vi "Periodic Tasks.vi"(8 "error in":errorcluster) -> ()   [LabVIEW 2018]
doc: "This VI runs in parallel to other tasks. It can contain as many user-defined periodic loops as you need. These can carry out PID or other sorts of timed response."
uses:
  <vilib>/Rock Robotics/WPI/DriverStation/WPI_DriverStationRobotMode2.ctl
  Cargo_motor_states.ctl
  control_states.ctl
  <vilib>/Rock Robotics/WPI/ThirdParty/Phoenix-LabVIEW/Motor Controller/Controls/CTRE_Phoenix_MotorControl_ControlMode.ctl
  GP_states.ctl
  <vilib>/Rock Robotics/WPI/Relay/WPI_RelayValue.ctl
  <vilib>/Analysis/baseanly.llb/Mean (DBL).vi
  <vilib>/Rock Robotics/Network Tables/NT Read Boolean.vi
  Robot Global Data.vi
  <vilib>/Rock Robotics/Network Tables/NT Read Numeric Array.vi
  <vilib>/Rock Robotics/Network Tables/NT Write Numeric Array.vi
  <vilib>/Rock Robotics/Network Tables/NT Write Boolean Array.vi
  <vilib>/Rock Robotics/Network Tables/NT Write Number.vi
  <vilib>/Rock Robotics/Network Tables/NT Read Number.vi
  <vilib>/addons/control/pid/pid.llb/PID (DBL).vi
  drivers/ADIS16470 IMU/ADIS16470_IMU.lvlib
  <vilib>/addons/control/pid/NI_PID_pid.lvlib
  <vilib>/Analysis/NI_AALBase.lvlib
panel:
  out "Robot Mode":T1
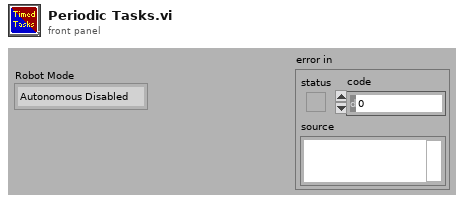
[diagram p1: front panel]
types:
  T1 = typedef "WPI_DriverStationRobotMode2.ctl" = enum16{"Autonomous Disabled", "Autonomous Enabled", "Teleop Disabled", "Teleop Enabled", "Disconnected", "Finish", "Test Disabled", "Test Enabled", "Emergency Stopped"}
  T2 = enum16{"open", "replace", "create", "open or create", "replace or create", "replace or create with confirmation"}
  T3 = typedef "Cargo_motor_states.ctl" = enum16{"Idle", "Intake", "Shoot"}
  T4 = typedef "ADIS16470_IMU.lvlib/ADI_IMU_ADIS16470_IMUDevRef.ctl" = cluster{"DevStatus":errorcluster, "Handle":i32, "SPI Bus":T5, "Device Found":bool, "Device Ready":bool, "Serial":u16, "Bytes Per Sample":u16, "Calibrate On Open?":bool}
  T5 = typedef "spi_bus.ctl" = enum16{"SPI On-Board, CS0", "SPI On-Board, CS1", "SPI On-Board, CS2", "SPI On-Board, CS3", "SPI MXP", "Invalid"}
  T6 = typedef "WPI_DigitalInputDevRef.ctl" = cluster{"DevStatus":errorcluster, "DIO Channel":T7}
  T7 = typedef "FPGA_DIOChannel.ctl" = enum8{"DIO 0", "DIO 1", "DIO 2", "DIO 3", "DIO 4", "DIO 5", "DIO 6", "DIO 7", "DIO 8", "DIO 9", "DIO MXP 0", "DIO MXP 1", "DIO MXP 2", "DIO MXP 3", "DIO MXP 4", "DIO MXP 5", "DIO MXP 6", "DIO MXP 7", "DIO MXP 8", "DIO MXP 9", "DIO MXP 10", "DIO MXP 11", "DIO MXP 12", "DIO MXP 13", "DIO MXP 14", "DIO MXP 15", "SPI Port CS1", "SPI Port CS2", "SPI Port CS3", "SPI Port MISO", "SPI Port MOSI", "Invalid"}
  T8 = typedef "WPI_PotentiometerDevRef.ctl" = cluster{"DevStatus":errorcluster, "Analog Channel":T9, "Invert Output":bool}
  T9 = typedef "FPGA_AIChannel.ctl" = enum8{"AI 0", "AI 1", "AI 2", "AI 3", "AI MXP 0", "AI MXP 1", "AI MXP 2", "AI MXP 3", "Invalid"}
  T10 = typedef "WPI_RelayDevRef.ctl" = cluster{"DevStatus":errorcluster, "Relay Channel":T11, "Relay Direction":T12}
  T11 = typedef "FPGA_DIORelayChannel.ctl" = enum8{"Relay 0", "Relay 1", "Relay 2", "Relay 3", "Invalid"}
  T12 = typedef "WPI_RelayDirection.ctl" = enum16{"Both directions", "Forward only", "Reverse only"}
  T13 = typedef "WPI_MotorControlDeviceRef.ctl" = cluster{"DeviceStatus":errorcluster, "Type":T14, "PWM":cluster{"PWM Channel":T15, "DeadBand":T16}, "CAN":cluster{"Device Number":u8, "SetOutput VI Ref":variant, "GetOutput VI Ref":variant, "Enable VI Ref":variant, "Disable VI Ref":variant, "Data":variant}, "Invert":bool, "DIO PWM":cluster{"PWM \"Enable\" Channel":T15, "DIOChannel":T7, "PWM Rate":dbl}}
  T14 = typedef "WPI_MotorControlType.ctl" = enum16{"PWM", "CAN", "DIO PWM"}
  T15 = typedef "FPGA_DIOPWMChannel.ctl" = enum8{"PWM 0", "PWM 1", "PWM 2", "PWM 3", "PWM 4", "PWM 5", "PWM 6", "PWM 7", "PWM 8", "PWM 9", "PWM MXP 0", "PWM MXP 1", "PWM MXP 2", "PWM MXP 3", "PWM MXP 4", "PWM MXP 5", "PWM MXP 6", "PWM MXP 7", "PWM MXP 8", "PWM MXP 9", "Invalid"}
  T16 = typedef "WPI_PWMDeadband.ctl" = cluster{"Name":string, "maxPositivePwm":i32, "minPositivePwm":i32, "centerPwm":i32, "maxNegativePwm":i32, "minNegativePwm":i32, "angularRange":u16}
  T17 = typedef "CTRE_Phoenix_MotorControl_ControlMode.ctl" = u16
  T18 = typedef "WPI_RelayValue.ctl" = enum16{"Off", "On", "Forward", "Reverse"}
  T19 = typedef "control_states.ctl" = enum16{"disable", "PID", "motor"}
  T20 = typedef "GP_states.ctl" = enum16{"Home", "AutoHome", "Hatch", "Ground"}
  T21 = cluster{"dorsalPID[0]":dbl, "dorsalPID[1]":dbl, "dorsalPID[2]":dbl}
  T22 = cluster{"fourbarPID[0]":dbl, "fourbarPID[1]":dbl, "fourbarPID[2]":dbl}
  T23 = cluster{"X Angle":dbl, "Y Angle":dbl, "Z Angle":dbl}
  T24 = cluster{"X Gyro":dbl, "Y Gyro":dbl, "Z Gyro":dbl, "X Accel":dbl, "Y Accel":dbl, "Z Accel":dbl, "Temp":dbl}
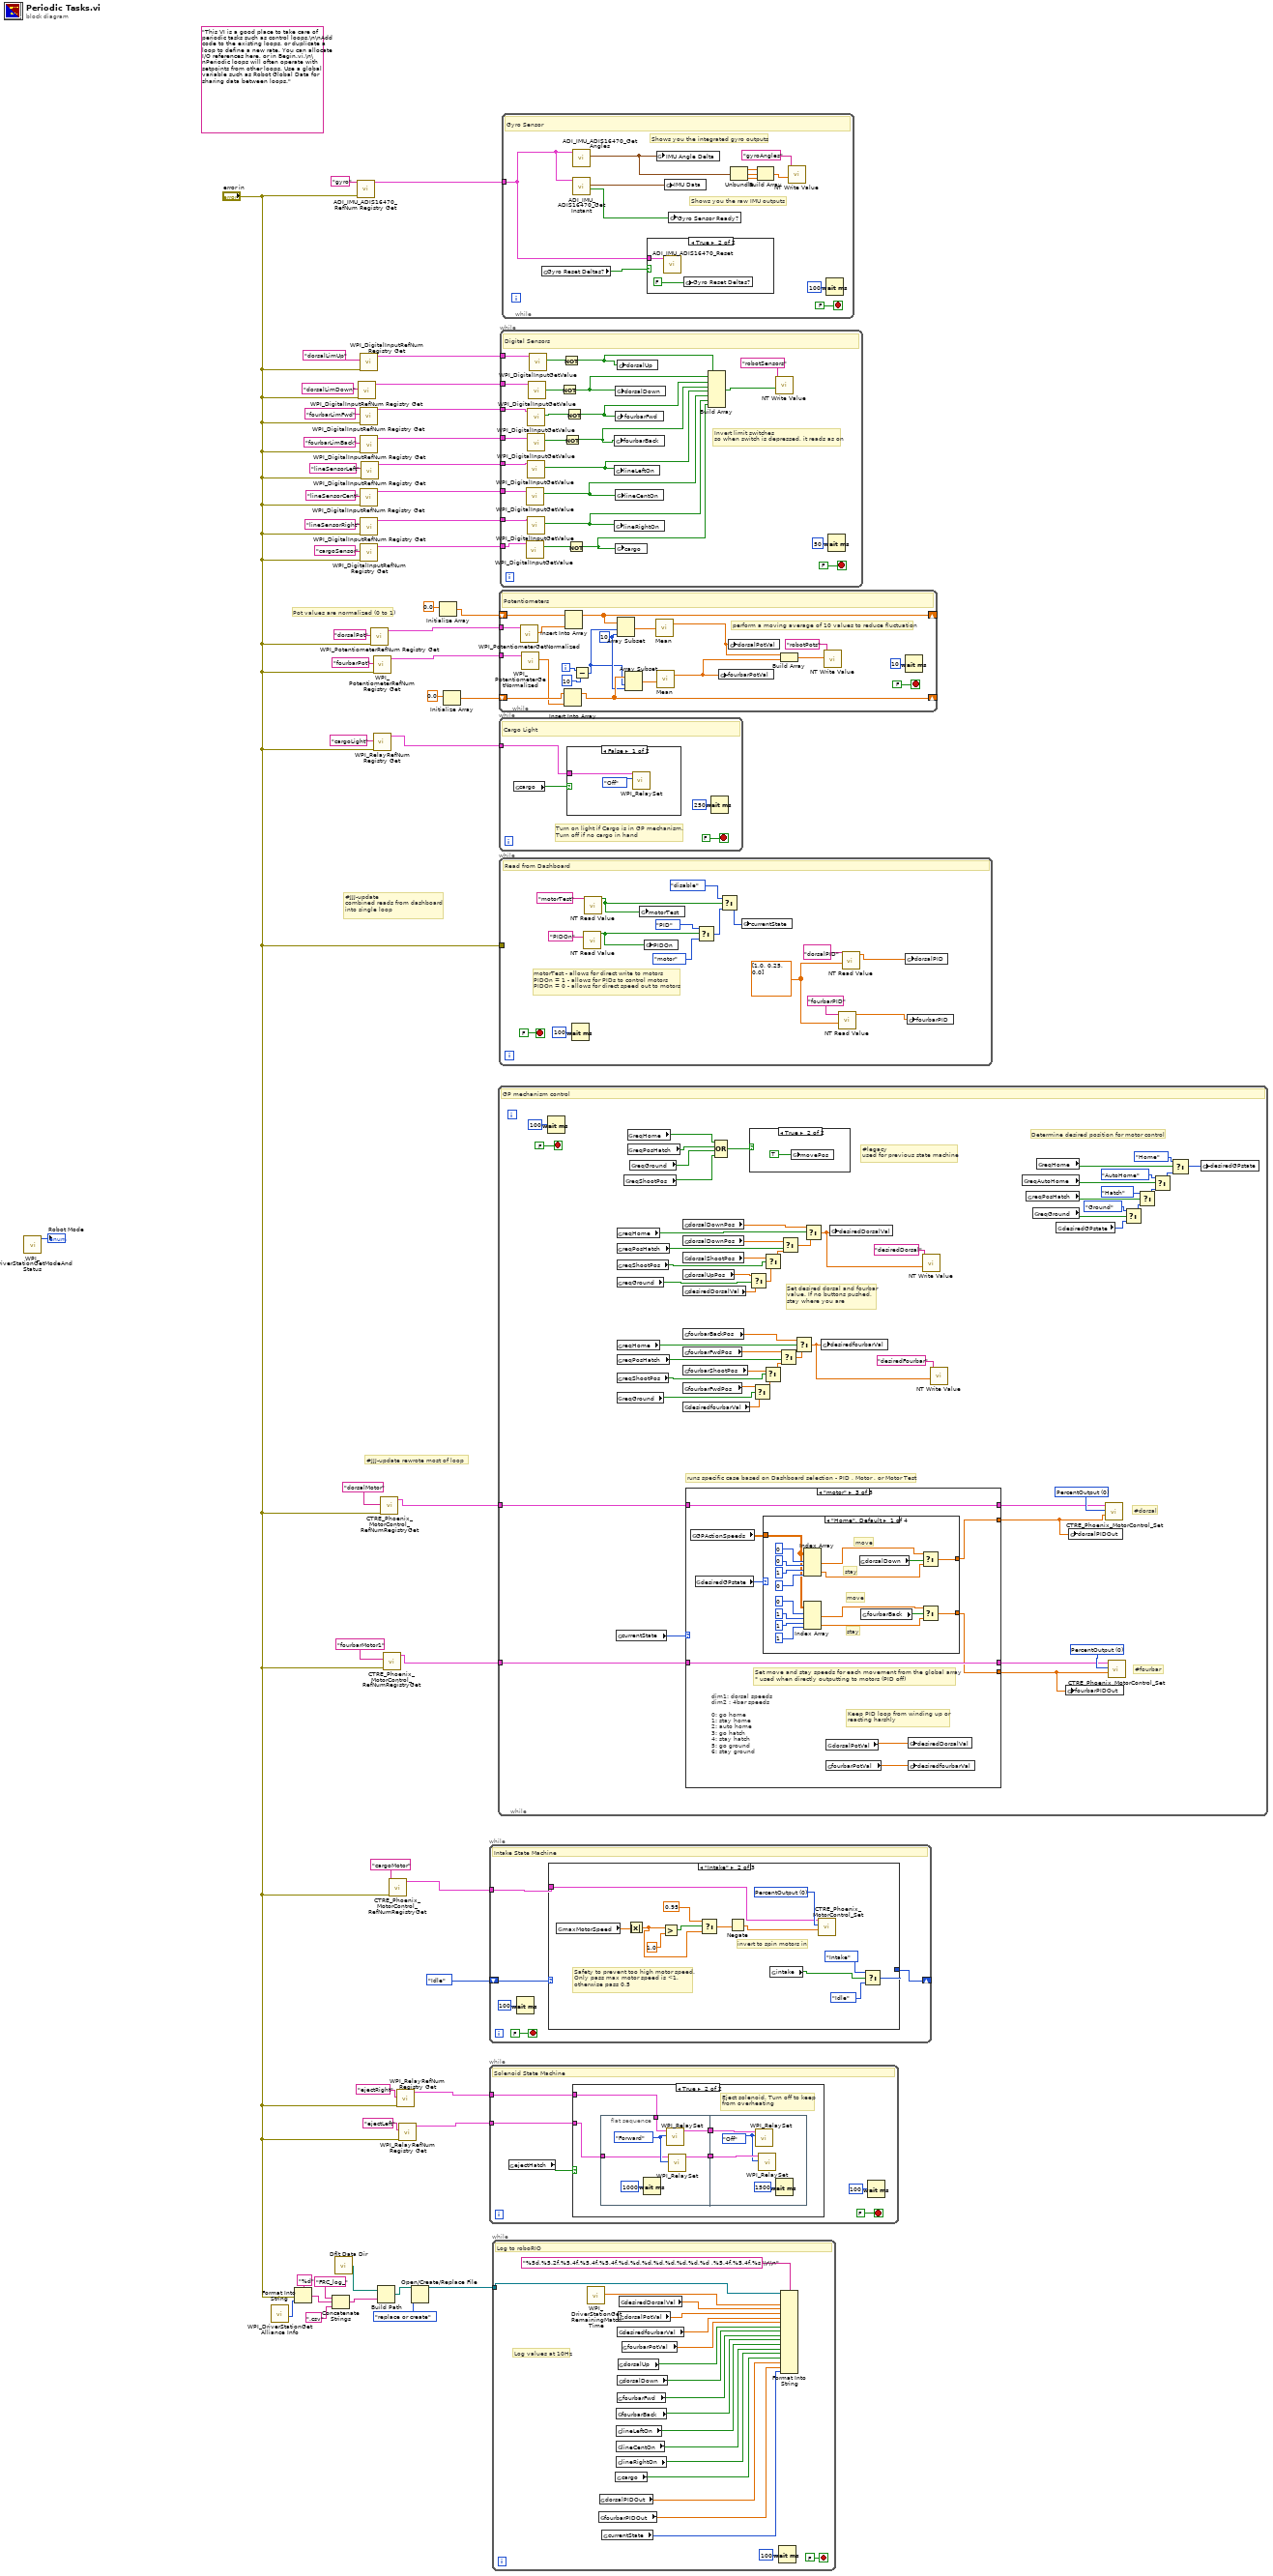
[diagram p0: block diagram]
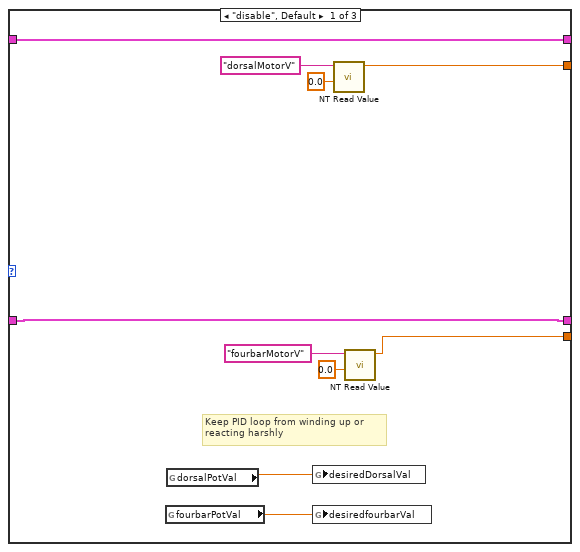
[diagram p2: hidden frame]
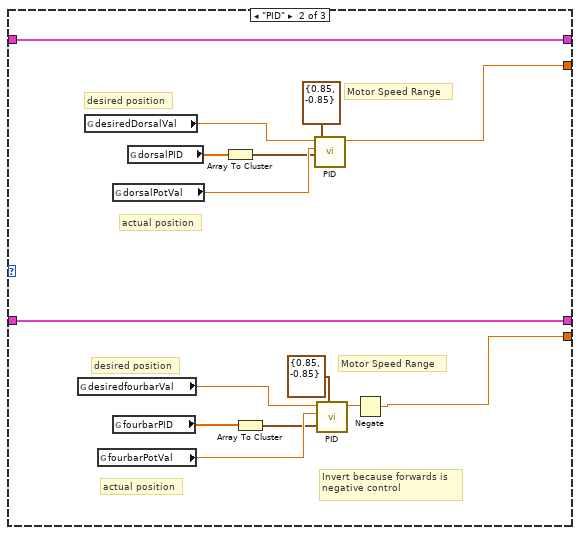
[diagram p3: hidden frame]
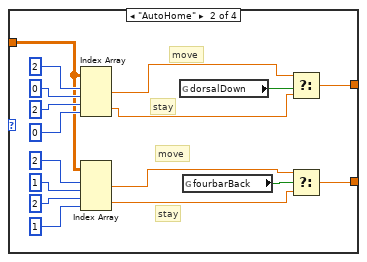
[diagram p4: hidden frame]
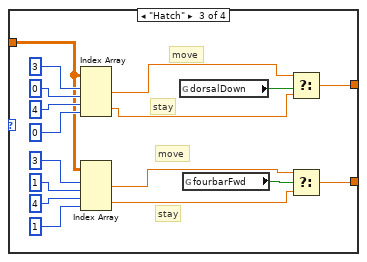
[diagram p5: hidden frame]
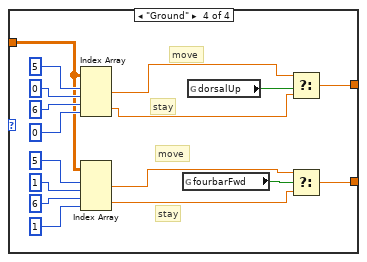
[diagram p6: hidden frame]
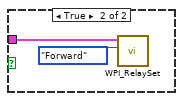
[diagram p8: hidden frame]
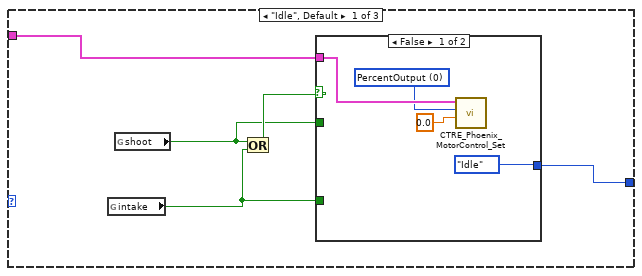
[diagram p10: hidden frame]
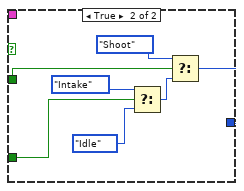
[diagram p11: hidden frame]
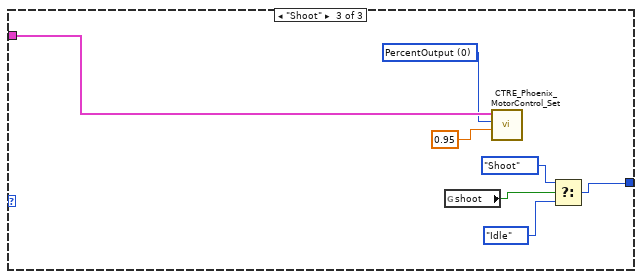
[diagram p12: hidden frame]
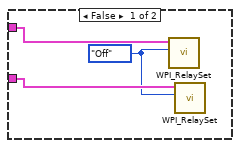
[diagram p13: hidden frame]
diagram:
  (unwired) "This VI is a good place to take care of periodic tasks such as control loops.\n\nAdd code to the existing loops, or duplicate a loop to define a new rate. You can allocate I/O references here, or in Begin.vi.\n\nPeriodic loops will often operate with setpoints from other loops. Use a global variable such as Robot Global Data for sharing data between loops."
  # "#JJJ-update rewrote most of loop"
  # "#JJJ-update\ncombined reads from dashboard\ninto single loop"
  # "Pot values are normalized (0 to 1)"
  n1 = call <vilib>:"WPI_DriverStationGetModeAndStatus.vi"() -> ("Robot Mode"=→"Robot Mode":T1)  [unwired: 10 in, 1 out]
  n2 = call <vilib>:"WPI_DriverStationGet Alliance Info.vi"() -> ("Match Number"=w9:u16)  [unwired: 6 in, 5 out]
  n3 = Format Into String(format string="%d", error in="error in", w9) -> (resulting string=w8:string)  [unwired: 1 in, 1 out]
  n4 = Concatenate Strings("FRC_log_", w8, ".csv" ("string")) -> (w12:string)
  n5 = call <vilib>:"Dflt Data Dir.vi"() -> ("App:Default Data Directory"=w16:path)
  n6 = call "ADI_IMU_ADIS16470_RefNum Registry Get.vi"("error in (no error)"="error in", "refnum name"="gyro") -> ("ADI IMU DevRef"=w51:T4)  [unwired: 8 in, 1 out]
  n7 = call <vilib>:"WPI_DigitalInputRefNum Registry Get.vi"("error in (no error)"="error in", "refnum name"="dorsalLimDown") -> ("DigitalInputDevRef"=w48:T6)  [unwired: 8 in, 1 out]
  n8 = call <vilib>:"WPI_DigitalInputRefNum Registry Get.vi"("error in (no error)"="error in", "refnum name"="dorsalLimUp") -> ("DigitalInputDevRef"=w49:T6)  [unwired: 8 in, 1 out]
  n9 = call <vilib>:"WPI_DigitalInputRefNum Registry Get.vi"("error in (no error)"="error in", "refnum name"="fourbarLimFwd") -> ("DigitalInputDevRef"=w47:T6)  [unwired: 8 in, 1 out]
  n10 = call <vilib>:"WPI_DigitalInputRefNum Registry Get.vi"("error in (no error)"="error in", "refnum name"="lineSensorCent") -> ("DigitalInputDevRef"=w44:T6)  [unwired: 8 in, 1 out]
  n11 = call <vilib>:"WPI_DigitalInputRefNum Registry Get.vi"("error in (no error)"="error in", "refnum name"="fourbarLimBack") -> ("DigitalInputDevRef"=w46:T6)  [unwired: 8 in, 1 out]
  n12 = call <vilib>:"WPI_DigitalInputRefNum Registry Get.vi"("error in (no error)"="error in", "refnum name"="lineSensorRight") -> ("DigitalInputDevRef"=w43:T6)  [unwired: 8 in, 1 out]
  n13 = call <vilib>:"WPI_DigitalInputRefNum Registry Get.vi"("error in (no error)"="error in", "refnum name"="cargoSensor") -> ("DigitalInputDevRef"=w42:T6)  [unwired: 8 in, 1 out]
  n14 = call <vilib>:"WPI_DigitalInputRefNum Registry Get.vi"("error in (no error)"="error in", "refnum name"="lineSensorLeft") -> ("DigitalInputDevRef"=w45:T6)  [unwired: 8 in, 1 out]
  n15 = call <vilib>:"WPI_PotentiometerRefNum Registry Get.vi"("error in (no error)"="error in", "refnum name"="dorsalPot") -> ("PotDevRef"=w40:T8)  [unwired: 8 in, 1 out]
  n16 = call <vilib>:"WPI_PotentiometerRefNum Registry Get.vi"("error in (no error)"="error in", "refnum name"="fourbarPot") -> ("PotDevRef"=w39:T8)  [unwired: 8 in, 1 out]
  n17 = call <vilib>:"WPI_RelayRefNum Registry Get.vi"("error in (no error)"="error in", "refnum name"="cargoLight") -> ("RelayDevRef"=w35:T10)  [unwired: 8 in, 1 out]
  n18 = Build Path(base path=w16, name or relative path=w12) -> (appended path=w15:path)
  n19 = call <vilib>:"CTRE_Phoenix_MotorControl_RefNumRegistryGet.vi"("error in (no error)"="error in", "refnum name"="dorsalMotor") -> ("PhoenixMotorControlDevRef"=w3:T13)  [unwired: 8 in, 1 out]
  n20 = call <vilib>:"CTRE_Phoenix_MotorControl_RefNumRegistryGet.vi"("error in (no error)"="error in", "refnum name"="fourbarMotor1") -> ("PhoenixMotorControlDevRef"=w5:T13)  [unwired: 8 in, 1 out]
  n21 = call <vilib>:"CTRE_Phoenix_MotorControl_RefNumRegistryGet.vi"("error in (no error)"="error in", "refnum name"="cargoMotor") -> ("PhoenixMotorControlDevRef"=w32:T13)  [unwired: 8 in, 1 out]
  n22 = call <vilib>:"WPI_RelayRefNum Registry Get.vi"("error in (no error)"="error in", "refnum name"="ejectRight") -> ("RelayDevRef"=w29:T10)  [unwired: 8 in, 1 out]
  n23 = call <vilib>:"WPI_RelayRefNum Registry Get.vi"("error in (no error)"="error in", "refnum name"="ejectLeft") -> ("RelayDevRef"=w28:T10)  [unwired: 8 in, 1 out]
  n24 = Open/Create/Replace File(file path (use dialog)=w15, operation (0:open)=T2."replace or create") -> (refnum out=w14:refnum<file>)  [unwired: 4 in, 2 out]
  n25 = Initialize Array(0.0 ("element")) -> (w27:dbl[])  [unwired: 1 in]
  n26 = Initialize Array(0.0 ("element")) -> (w24:dbl[])  [unwired: 1 in]
  n27 = while {
    tunnel: w32 -> [w54]
    shift-right: [w52] -> _
    shift-left: Cargo_motor_states."Idle" ("Enum") -> [w55]
    stop <- FALSE stop-if-true
    # "Intake State Machine"
    n28 = Wait (ms)(milliseconds to wait=u32 100) -> ()  [unwired: 1 out]
    n29 = case shown="\"Intake\"" w55 {
      tunnel: w54 -> [w60 w75 w92]
      tunnel: [w59 w78 w87] -> w52
      frame "Idle", Default {
        n30 = global read "Robot Global Data.vi" "intake"() -> (w57:bool)
        n31 = global read "Robot Global Data.vi" "shoot"() -> (w58:bool)
        n32 = Or(x=w58, y=w57) -> (x .or. y?=w61:bool)
        n33 = case shown="False" w61 {
          tunnel: w60 -> [w65 _]
          tunnel: [Cargo_motor_states."Idle" ("Enum") w70] -> w59
          tunnel: w58 -> [_ w71]
          tunnel: w57 -> [_ w66]
          frame False {
            w64 = T17 0 items=["PercentOutput"=0, "Position"=1, "Velocity"=2, "Current"=3, "Follower"=5, "MotionProfile"=6, "MotionMagic"=7, "MotionProfileArc"=10, "Disabled"=15] ("Control Mode")
            n34 = call <vilib>:"CTRE_Phoenix_MotorControl_Set.vi"("Output"=0.0, "Control Mode"=w64, "PhoenixMotorControlDevRef"=w65) -> ()  [unwired: 7 in, 2 out]
          }
          frame True {
            n35 = Select(t=Cargo_motor_states."Intake" ("Enum"), s=w66, f=Cargo_motor_states."Idle" ("Enum")) -> (s? t:f=w72:T3)
            n36 = Select(t=Cargo_motor_states."Shoot" ("Enum"), s=w71, f=w72) -> (s? t:f=w70:T3)
          }
        }
      }
      frame "Intake" {
        w77 = T17 0 items=["PercentOutput"=0, "Position"=1, "Velocity"=2, "Current"=3, "Follower"=5, "MotionProfile"=6, "MotionMagic"=7, "MotionProfileArc"=10, "Disabled"=15] ("Control Mode")
        # "invert to spin motors in"
        # "Safety to prevent too high motor speed.\nOnly pass max motor speed is <1, \notherwise pass 0.5"
        n37 = global read "Robot Global Data.vi" "maxMotorSpeed"() -> (w85:dbl)
        n38 = Absolute Value(x=w85) -> (abs(x)=w74:dbl)
        n39 = Greater?(x=w74, y=1.0) -> (0:w83:bool)
        n40 = Select(t=0.95, s=w83, f=w74) -> (s? t:f=w81:dbl)
        n41 = Negate(x=w81) -> (-x=w76:dbl)
        n42 = global read "Robot Global Data.vi" "intake"() -> (w73:bool)
        n43 = call <vilib>:"CTRE_Phoenix_MotorControl_Set.vi"("Output"=w76, "Control Mode"=w77, "PhoenixMotorControlDevRef"=w75) -> ()  [unwired: 7 in, 2 out]
        n44 = Select(t=Cargo_motor_states."Intake" ("Enum"), s=w73, f=Cargo_motor_states."Idle" ("Enum")) -> (s? t:f=w78:T3)
      }
      frame "Shoot" {
        w91 = T17 0 items=["PercentOutput"=0, "Position"=1, "Velocity"=2, "Current"=3, "Follower"=5, "MotionProfile"=6, "MotionMagic"=7, "MotionProfileArc"=10, "Disabled"=15] ("Control Mode")
        n45 = global read "Robot Global Data.vi" "shoot"() -> (w90:bool)
        n46 = call <vilib>:"CTRE_Phoenix_MotorControl_Set.vi"("Output"=0.95, "Control Mode"=w91, "PhoenixMotorControlDevRef"=w92) -> ()  [unwired: 7 in, 2 out]
        n47 = Select(t=Cargo_motor_states."Shoot" ("Enum"), s=w90, f=Cargo_motor_states."Idle" ("Enum")) -> (s? t:f=w87:T3)
      }
    }
  }
  n48 = while {
    tunnel: w29 -> [w95]
    tunnel: w28 -> [w94]
    stop <- FALSE stop-if-true
    # "Solenoid State Machine"
    n49 = global read "Robot Global Data.vi" "ejectHatch"() -> (w97:bool)
    n50 = case shown="True" w97 {
      tunnel: w95 -> [w100 w103]
      tunnel: w94 -> [w99 w104]
      frame False {
        w98 = WPI_RelayValue."Off" ("RelayValue")
        n51 = call <vilib>:"WPI_RelaySet.vi"("RelayValue"=w98, "RelayDevRef"=w100) -> ()  [unwired: 8 in, 2 out]
        n52 = call <vilib>:"WPI_RelaySet.vi"("RelayValue"=w98, "RelayDevRef"=w99) -> ()  [unwired: 8 in, 2 out]
      }
      frame True {
        # "Eject solenoid. Turn off to keep\nfrom overheating"
        n53 = flat-sequence {
          tunnel: w104 -> [w109]
          tunnel: w103 -> [w108]
          tunnel: [w106] -> w102
          tunnel: [w105] -> w101
          tunnel: w102 -> [w114]
          tunnel: w101 -> [w113]
          frame #0 {
            w110 = WPI_RelayValue."Forward" ("RelayValue")
            n54 = Wait (ms)(milliseconds to wait=u32 1000) -> ()  [unwired: 1 out]
            n55 = call <vilib>:"WPI_RelaySet.vi"("RelayValue"=w110, "RelayDevRef"=w108) -> ("RelayDevRef"=w106:T10)  [unwired: 8 in, 1 out]
            n56 = call <vilib>:"WPI_RelaySet.vi"("RelayValue"=w110, "RelayDevRef"=w109) -> ("RelayDevRef"=w105:T10)  [unwired: 8 in, 1 out]
          }
          frame #1 {
            w112 = WPI_RelayValue."Off" ("RelayValue")
            n57 = call <vilib>:"WPI_RelaySet.vi"("RelayValue"=w112, "RelayDevRef"=w114) -> ()  [unwired: 8 in, 2 out]
            n58 = call <vilib>:"WPI_RelaySet.vi"("RelayValue"=w112, "RelayDevRef"=w113) -> ()  [unwired: 8 in, 2 out]
            n59 = Wait (ms)(milliseconds to wait=u32 1500) -> ()  [unwired: 1 out]
          }
        }
      }
    }
    n60 = Wait (ms)(milliseconds to wait=u32 100) -> ()  [unwired: 1 out]
  }
  n61 = while {
    tunnel: w14 -> [w127]
    stop <- FALSE stop-if-true
    # "Log values at 10Hz"
    # "Log to roboRIO"
    n62 = call <vilib>:"WPI_DriverStationGetRemainingMatchTime.vi"() -> ("Match Time(s)"=w126:sgl)  [unwired: 10 in, 1 out]
    n63 = global read "Robot Global Data.vi" "fourbarPIDOut"() -> (w116:dbl)
    n64 = global read "Robot Global Data.vi" "dorsalPIDOut"() -> (w117:dbl)
    n65 = global read "Robot Global Data.vi" "currentState"() -> (w115:T19)
    n66 = global read "Robot Global Data.vi" "cargo"() -> (w118:bool)
    n67 = global read "Robot Global Data.vi" "fourbarBack"() -> (w122:bool)
    n68 = global read "Robot Global Data.vi" "lineLeftOn"() -> (w121:bool)
    n69 = global read "Robot Global Data.vi" "lineCentOn"() -> (w120:bool)
    n70 = global read "Robot Global Data.vi" "lineRightOn"() -> (w119:bool)
    n71 = global read "Robot Global Data.vi" "fourbarFwd"() -> (w123:bool)
    n72 = global read "Robot Global Data.vi" "desiredfourbarVal"() -> (w131:dbl)
    n73 = global read "Robot Global Data.vi" "dorsalDown"() -> (w124:bool)
    n74 = global read "Robot Global Data.vi" "dorsalUp"() -> (w125:bool)
    n75 = global read "Robot Global Data.vi" "dorsalPotVal"() -> (w132:dbl)
    n76 = global read "Robot Global Data.vi" "desiredDorsalVal"() -> (w133:dbl)
    n77 = global read "Robot Global Data.vi" "fourbarPotVal"() -> (w130:dbl)
    n78 = Wait (ms)(milliseconds to wait=u32 100) -> ()  [unwired: 1 out]
    n79 = Format Into String(format string="%5d,%5.2f,%5.4f,%5.4f,%5.4f,%d,%d,%d,%d,%d,%d,%d,%d ,%5.4f,%5.4f,%s \\r\\n", initial string=w127, w126, w133, w132, w131, w130, w125, w124, w123, w122, w121, w120, w119, w118, w117, w116, w115) -> ()  [unwired: 1 in, 2 out]
  }
  n80 = while {
    tunnel: w5 -> [w151]
    tunnel: w3 -> [w154]
    stop <- FALSE stop-if-true
    w155 = T17 0 items=["PercentOutput"=0, "Position"=1, "Velocity"=2, "Current"=3, "Follower"=5, "MotionProfile"=6, "MotionMagic"=7, "MotionProfileArc"=10, "Disabled"=15] ("Control Mode")
    w156 = T17 0 items=["PercentOutput"=0, "Position"=1, "Velocity"=2, "Current"=3, "Follower"=5, "MotionProfile"=6, "MotionMagic"=7, "MotionProfileArc"=10, "Disabled"=15] ("Control Mode")
    # "Determine desired position for motor control"
    # "runs specific case based on Dashboard selection - PID , Motor , or Motor Test"
    # "#legacy\nused for previous state machine"
    # "#fourbar"
    # "#dorsal"
    # "Set desired dorsal and fourbar\nvalue. If no buttons pushed,\nstay where you are"
    # "GP mechanism control"
    n81 = Wait (ms)(milliseconds to wait=u32 100) -> ()  [unwired: 1 out]
    n82 = global read "Robot Global Data.vi" "currentState"() -> (w150:T19)
    n83 = global read "Robot Global Data.vi" "reqHome"() -> (w189:bool)
    n84 = global read "Robot Global Data.vi" "reqPosHatch"() -> (w188:bool)
    n85 = global read "Robot Global Data.vi" "reqShootPos"() -> (w186:bool)
    n86 = global read "Robot Global Data.vi" "reqGround"() -> (w184:bool)
    n87 = global read "Robot Global Data.vi" "reqHome"() -> (w178:bool)
    n88 = global read "Robot Global Data.vi" "reqPosHatch"() -> (w177:bool)
    n89 = global read "Robot Global Data.vi" "reqShootPos"() -> (w175:bool)
    n90 = global read "Robot Global Data.vi" "reqGround"() -> (w173:bool)
    n91 = global read "Robot Global Data.vi" "reqShootPos"() -> (w164:bool)
    n92 = global read "Robot Global Data.vi" "reqHome"() -> (w161:bool)
    n93 = global read "Robot Global Data.vi" "reqPosHatch"() -> (w162:bool)
    n94 = global read "Robot Global Data.vi" "reqGround"() -> (w163:bool)
    n95 = global read "Robot Global Data.vi" "dorsalDownPos"() -> (w182:dbl)
    n96 = global read "Robot Global Data.vi" "dorsalDownPos"() -> (w181:dbl)
    n97 = global read "Robot Global Data.vi" "dorsalShootPos"() -> (w180:dbl)
    n98 = global read "Robot Global Data.vi" "dorsalUpPos"() -> (w179:dbl)
    n99 = global read "Robot Global Data.vi" "desiredDorsalVal"() -> (w167:dbl)
    n100 = global read "Robot Global Data.vi" "fourbarBackPos"() -> (w171:dbl)
    n101 = global read "Robot Global Data.vi" "fourbarFwdPos"() -> (w170:dbl)
    n102 = global read "Robot Global Data.vi" "fourbarShootPos"() -> (w169:dbl)
    n103 = global read "Robot Global Data.vi" "fourbarFwdPos"() -> (w168:dbl)
    n104 = global read "Robot Global Data.vi" "desiredfourbarVal"() -> (w166:dbl)
    n105 = case shown="\"motor\"" w150 {
      tunnel: w154 -> [w197 w205 w222]
      tunnel: [w197 w205 w222] -> w153
      tunnel: [w196 w204 w221] -> w152
      tunnel: w151 -> [w196 w204 w221]
      tunnel: [w193 w203 w219] -> w149
      tunnel: [w192 w202 w218] -> w148
      frame "disable", Default {
        # "Keep PID loop from winding up or\nreacting harshly"
        n106 = global read "Robot Global Data.vi" "fourbarPotVal"() -> (w195:dbl)
        n107 = global read "Robot Global Data.vi" "dorsalPotVal"() -> (w194:dbl)
        n108 = global write "Robot Global Data.vi" "desiredDorsalVal"(w194) -> ()
        n109 = global write "Robot Global Data.vi" "desiredfourbarVal"(w195) -> ()
        n110 = call-poly <vilib>:"NT Read Value.vi"("Default Value"=0.0, "Name"="dorsalMotorV" ("refnum name")) -> ("Numeric"=w193:dbl)  [unwired: 8 in, 1 out]
        n111 = call-poly <vilib>:"NT Read Value.vi"("Default Value"=0.0, "Name"="fourbarMotorV" ("refnum name")) -> ("Numeric"=w192:dbl)  [unwired: 8 in, 1 out]
      }
      frame "PID" {
        # "Invert because forwards is \nnegative control"
        # "actual position"
        # "desired position"
        # "Motor Speed Range"
        # "actual position"
        # "desired position"
        # "Motor Speed Range"
        n112 = global read "Robot Global Data.vi" "desiredfourbarVal"() -> (w209:dbl)
        n113 = global read "Robot Global Data.vi" "desiredDorsalVal"() -> (w215:dbl)
        n114 = global read "Robot Global Data.vi" "fourbarPotVal"() -> (w212:dbl)
        n115 = global read "Robot Global Data.vi" "dorsalPotVal"() -> (w214:dbl)
        n116 = global read "Robot Global Data.vi" "fourbarPID"() -> (w206:dbl[])
        n117 = global read "Robot Global Data.vi" "dorsalPID"() -> (w207:dbl[])
        n118 = Array To Cluster(array=w207) -> (cluster=w213:T21)
        n119 = Array To Cluster(array=w206) -> (cluster=w211:T22)
        n120 = call-poly <vilib>:"PID.vi"("output range"=cluster{"output high":dbl, "output low":dbl} {"output high"=0.85, "output low"=-0.85}, "PID gains"=w213, "process variable"=w214, "setpoint"=w215) -> ("output"=w203:dbl)  [unwired: 6 in, 1 out]
        n121 = call-poly <vilib>:"PID.vi"("output range"=cluster{"output high":dbl, "output low":dbl} {"output high"=0.85, "output low"=-0.85}, "PID gains"=w211, "process variable"=w212, "setpoint"=w209) -> ("output"=w210:dbl)  [unwired: 6 in, 1 out]
        n122 = Negate(x=w210) -> (-x=w202:dbl)
      }
      frame "motor" {
        # "Set move and stay speeds for each movement from the global array\n* used when directly outputting to motors (PID off)"
        # "dim1: dorsal speeds\ndim2 : 4bar speeds\n\n0: go home\n1: stay home\n2: auto home\n3: go hatch\n4: stay hatch\n5: go ground\n6: stay ground"
        # "Keep PID loop from winding up or\nreacting harshly"
        n123 = global read "Robot Global Data.vi" "GPActionSpeeds"() -> (w217:dbl[][])
        n124 = global read "Robot Global Data.vi" "desiredGPstate"() -> (w220:T20)
        n125 = case shown="\"Home\", Default" w220 {
          tunnel: [w241 w258 w275 w292] -> w219
          tunnel: [w240 w257 w274 w291] -> w218
          tunnel: w217 -> [w225 w242 w259 w276]
          frame "Home", Default {
            # "stay"
            # "move"
            # "stay"
            # "move"
            n126 = Index Array(array=w225, index (row) #1=0 ("disabled index (col)"), index (col) #1=0 ("disabled index (col)"), index (row) #2=1 ("disabled index (col)"), index (col) #2=0 ("disabled index (col)")) -> (element #1=w236:dbl, element #2=w235:dbl)
            n127 = Index Array(array=w225, index (row) #1=0 ("disabled index (col)"), index (col) #1=1 ("disabled index (col)"), index (row) #2=1 ("disabled index (col)"), index (col) #2=1 ("disabled index (col)")) -> (element #1=w227:dbl, element #2=w226:dbl)
            n128 = global read "Robot Global Data.vi" "dorsalDown"() -> (w238:bool)
            n129 = global read "Robot Global Data.vi" "fourbarBack"() -> (w239:bool)
            n130 = Select(t=w236, s=w238, f=w235) -> (s? t:f=w241:dbl)
            n131 = Select(t=w227, s=w239, f=w226) -> (s? t:f=w240:dbl)
          }
          frame "AutoHome" {
            # "stay"
            # "move"
            # "stay"
            # "move"
            n132 = Index Array(array=w242, index (row) #1=2 ("disabled index (col)"), index (col) #1=0 ("disabled index (col)"), index (row) #2=2 ("disabled index (col)"), index (col) #2=0 ("disabled index (col)")) -> (element #1=w253:dbl, element #2=w252:dbl)
            n133 = Index Array(array=w242, index (row) #1=2 ("disabled index (col)"), index (col) #1=1 ("disabled index (col)"), index (row) #2=2 ("disabled index (col)"), index (col) #2=1 ("disabled index (col)")) -> (element #1=w244:dbl, element #2=w243:dbl)
            n134 = global read "Robot Global Data.vi" "dorsalDown"() -> (w255:bool)
            n135 = global read "Robot Global Data.vi" "fourbarBack"() -> (w256:bool)
            n136 = Select(t=w253, s=w255, f=w252) -> (s? t:f=w258:dbl)
            n137 = Select(t=w244, s=w256, f=w243) -> (s? t:f=w257:dbl)
          }
          frame "Hatch" {
            # "stay"
            # "move"
            # "stay"
            # "move"
            n138 = Index Array(array=w259, index (row) #1=3 ("disabled index (col)"), index (col) #1=0 ("disabled index (col)"), index (row) #2=4 ("disabled index (col)"), index (col) #2=0 ("disabled index (col)")) -> (element #1=w270:dbl, element #2=w269:dbl)
            n139 = Index Array(array=w259, index (row) #1=3 ("disabled index (col)"), index (col) #1=1 ("disabled index (col)"), index (row) #2=4 ("disabled index (col)"), index (col) #2=1 ("disabled index (col)")) -> (element #1=w261:dbl, element #2=w260:dbl)
            n140 = global read "Robot Global Data.vi" "dorsalDown"() -> (w272:bool)
            n141 = global read "Robot Global Data.vi" "fourbarFwd"() -> (w273:bool)
            n142 = Select(t=w270, s=w272, f=w269) -> (s? t:f=w275:dbl)
            n143 = Select(t=w261, s=w273, f=w260) -> (s? t:f=w274:dbl)
          }
          frame "Ground" {
            # "stay"
            # "move"
            # "stay"
            # "move"
            n144 = Index Array(array=w276, index (row) #1=5 ("disabled index (col)"), index (col) #1=0 ("disabled index (col)"), index (row) #2=6 ("disabled index (col)"), index (col) #2=0 ("disabled index (col)")) -> (element #1=w287:dbl, element #2=w286:dbl)
            n145 = Index Array(array=w276, index (row) #1=5 ("disabled index (col)"), index (col) #1=1 ("disabled index (col)"), index (row) #2=6 ("disabled index (col)"), index (col) #2=1 ("disabled index (col)")) -> (element #1=w278:dbl, element #2=w277:dbl)
            n146 = global read "Robot Global Data.vi" "fourbarFwd"() -> (w290:bool)
            n147 = global read "Robot Global Data.vi" "dorsalUp"() -> (w289:bool)
            n148 = Select(t=w287, s=w289, f=w286) -> (s? t:f=w292:dbl)
            n149 = Select(t=w278, s=w290, f=w277) -> (s? t:f=w291:dbl)
          }
        }
        n150 = global read "Robot Global Data.vi" "fourbarPotVal"() -> (w224:dbl)
        n151 = global read "Robot Global Data.vi" "dorsalPotVal"() -> (w223:dbl)
        n152 = global write "Robot Global Data.vi" "desiredDorsalVal"(w223) -> ()
        n153 = global write "Robot Global Data.vi" "desiredfourbarVal"(w224) -> ()
      }
    }
    n154 = Compound Arithmetic op=OR(w161, w162, w163, w164) -> (w165:bool)
    n155 = case shown="True" w165 {
      frame False {
      }
      frame True {
        n156 = global write "Robot Global Data.vi" "movePos"(TRUE ("movePos")) -> ()
      }
    }
    n157 = Select(t=w179, s=w184, f=w167) -> (s? t:f=w183:dbl)
    n158 = Select(t=w168, s=w173, f=w166) -> (s? t:f=w172:dbl)
    n159 = Select(t=w169, s=w175, f=w172) -> (s? t:f=w174:dbl)
    n160 = Select(t=w180, s=w186, f=w183) -> (s? t:f=w185:dbl)
    n161 = Select(t=w170, s=w177, f=w174) -> (s? t:f=w176:dbl)
    n162 = Select(t=w181, s=w188, f=w185) -> (s? t:f=w187:dbl)
    n163 = Select(t=w171, s=w178, f=w176) -> (s? t:f=w157:dbl)
    n164 = Select(t=w182, s=w189, f=w187) -> (s? t:f=w159:dbl)
    n165 = global write "Robot Global Data.vi" "desiredfourbarVal"(w157) -> ()
    n166 = global write "Robot Global Data.vi" "desiredDorsalVal"(w159) -> ()
    n167 = call-poly <vilib>:"NT Write Value.vi"("Numeric"=w159, "Name"="desiredDorsal") -> ()  [unwired: 9 in, 1 out]
    n168 = call-poly <vilib>:"NT Write Value.vi"("Numeric"=w157, "Name"="desiredFourbar") -> ()  [unwired: 9 in, 1 out]
    n169 = global read "Robot Global Data.vi" "reqAutoHome"() -> (w145:bool)
    n170 = global read "Robot Global Data.vi" "reqPosHatch"() -> (w144:bool)
    n171 = global read "Robot Global Data.vi" "reqGround"() -> (w141:bool)
    n172 = global read "Robot Global Data.vi" "reqHome"() -> (w147:bool)
    n173 = global read "Robot Global Data.vi" "desiredGPstate"() -> (w135:T20)
    n174 = global write "Robot Global Data.vi" "fourbarPIDOut"(w148) -> ()
    n175 = global write "Robot Global Data.vi" "dorsalPIDOut"(w149) -> ()
    n176 = call <vilib>:"CTRE_Phoenix_MotorControl_Set.vi"("Output"=w149, "Control Mode"=w156, "PhoenixMotorControlDevRef"=w153) -> ()  [unwired: 7 in, 2 out]
    n177 = call <vilib>:"CTRE_Phoenix_MotorControl_Set.vi"("Output"=w148, "Control Mode"=w155, "PhoenixMotorControlDevRef"=w152) -> ()  [unwired: 7 in, 2 out]
    n178 = Select(t=GP_states."Ground" ("GP_states"), s=w141, f=w135) -> (s? t:f=w143:T20)
    n179 = Select(t=GP_states."Hatch" ("GP_states"), s=w144, f=w143) -> (s? t:f=w142:T20)
    n180 = Select(t=GP_states."AutoHome" ("GP_states"), s=w145, f=w142) -> (s? t:f=w146:T20)
    n181 = Select(t=GP_states."Home" ("GP_states"), s=w147, f=w146) -> (s? t:f=w137:T20)
    n182 = global write "Robot Global Data.vi" "desiredGPstate"(w137) -> ()
  }
  n183 = while {
    tunnel: w40 -> [w313]
    tunnel: w39 -> [w310]
    shift-right: [w305] -> _
    shift-left: w27 -> [w307]
    shift-right: [w298] -> _
    shift-left: w24 -> [w300]
    i -> [w304]
    stop <- FALSE stop-if-true
    w297 = 10 ("length")
    # "perform a moving average of 10 values to reduce fluctuation"
    # "Potentiometers"
    n184 = call <vilib>:"WPI_PotentiometerGetNormalized.vi"("PotDevRef"=w313) -> ("Normalized Value"=w306:dbl)  [unwired: 8 in, 2 out]
    n185 = call <vilib>:"WPI_PotentiometerGetNormalized.vi"("PotDevRef"=w310) -> ("Normalized Value"=w299:dbl)  [unwired: 8 in, 2 out]
    n186 = Insert Into Array(array=w300, new element=w299) -> (w298:dbl[])  [unwired: 1 in]
    n187 = Insert Into Array(array=w307, new element=w306) -> (w305:dbl[])  [unwired: 1 in]
    n188 = Subtract(x=w304, y=10) -> (x-y=w296:i32)
    n189 = Array Subset(array=w305, index=w296, length=w297) -> (w303:dbl[])
    n190 = Array Subset(array=w298, index=w296, length=w297) -> (w295:dbl[])
    n191 = call-poly <vilib>:"Mean.vi"("X"=w303) -> ("mean"=w302:dbl)  [unwired: 1 out]
    n192 = call-poly <vilib>:"Mean.vi"("X"=w295) -> ("mean"=w294:dbl)  [unwired: 1 out]
    n193 = global write "Robot Global Data.vi" "fourbarPotVal"(w294) -> ()
    n194 = global write "Robot Global Data.vi" "dorsalPotVal"(w302) -> ()
    n195 = Build Array(w302, w294) -> (w309:dbl[])
    n196 = call-poly <vilib>:"NT Write Value.vi"("Numeric Array"=w309, "Name"="robotPots") -> ()  [unwired: 9 in, 1 out]
    n197 = Wait (ms)(milliseconds to wait=u32 10) -> ()  [unwired: 1 out]
  }
  n198 = while {
    tunnel: w35 -> [w314]
    stop <- FALSE stop-if-true
    # "Turn on light if Cargo is in GP mechanism.\nTurn off if no cargo in hand"
    # "Cargo Light"
    n199 = global read "Robot Global Data.vi" "cargo"() -> (w315:bool)
    n200 = case shown="False" w315 {
      tunnel: w314 -> [w318 w321]
      frame False {
        n201 = call <vilib>:"WPI_RelaySet.vi"("RelayValue"=WPI_RelayValue."Off", "RelayDevRef"=w318) -> ()  [unwired: 8 in, 2 out]
      }
      frame True {
        n202 = call <vilib>:"WPI_RelaySet.vi"("RelayValue"=WPI_RelayValue."Forward", "RelayDevRef"=w321) -> ()  [unwired: 8 in, 2 out]
      }
    }
    n203 = Wait (ms)(milliseconds to wait=u32 250) -> ()  [unwired: 1 out]
  }
  n204 = while {
    tunnel: "error in" -> [_]
    stop <- FALSE stop-if-true
    w332 = dbl[] [1.0, 0.25, 0.0] ("Default Value")
    # "motorTest - allows for direct write to motors\nPIDOn = 1 - allows for PIDs to control motors\nPIDOn = 0 - allows for direct speed out to motors"
    # "Read from Dashboard"
    n205 = Wait (ms)(milliseconds to wait=u32 100) -> ()  [unwired: 1 out]
    n206 = call-poly <vilib>:"NT Read Value.vi"("Name"="PIDOn") -> ("Boolean"=w325:bool)  [unwired: 9 in, 1 out]
    n207 = call-poly <vilib>:"NT Read Value.vi"("Name"="motorTest") -> ("Boolean"=w328:bool)  [unwired: 9 in, 1 out]
    n208 = global write "Robot Global Data.vi" "motorTest"(w328) -> ()
    n209 = global write "Robot Global Data.vi" "PIDOn"(w325) -> ()
    n210 = Select(t=control_states."PID" ("Enum"), s=w325, f=control_states."motor" ("Enum")) -> (s? t:f=w324:T19)
    n211 = Select(t=control_states."disable" ("Enum"), s=w328, f=w324) -> (s? t:f=w326:T19)
    n212 = global write "Robot Global Data.vi" "currentState"(w326) -> ()
    n213 = call-poly <vilib>:"NT Read Value.vi"("Default Value"=w332, "Name"="fourbarPID") -> ("Numeric Array"=w333:dbl[])  [unwired: 8 in, 1 out]
    n214 = call-poly <vilib>:"NT Read Value.vi"("Default Value"=w332, "Name"="dorsalPID") -> ("Numeric Array"=w329:dbl[])  [unwired: 8 in, 1 out]
    n215 = global write "Robot Global Data.vi" "dorsalPID"(w329) -> ()
    n216 = global write "Robot Global Data.vi" "fourbarPID"(w333) -> ()
  }
  n217 = while {
    tunnel: w49 -> [w361]
    tunnel: w48 -> [w360]
    tunnel: w47 -> [w359]
    tunnel: w46 -> [w358]
    tunnel: w45 -> [w355]
    tunnel: w44 -> [w354]
    tunnel: w43 -> [w353]
    tunnel: w42 -> [w352]
    stop <- FALSE stop-if-true
    # "Invert limit switches \nso when switch is depressed, it reads as on"
    # "Digital Sensors"
    n218 = call <vilib>:"WPI_DigitalInputGetValue.vi"("DigitalInputDevRef"=w352) -> ("Value"=w343:bool)  [unwired: 8 in, 2 out]
    n219 = call <vilib>:"WPI_DigitalInputGetValue.vi"("DigitalInputDevRef"=w354) -> ("Value"=w350:bool)  [unwired: 8 in, 2 out]
    n220 = call <vilib>:"WPI_DigitalInputGetValue.vi"("DigitalInputDevRef"=w355) -> ("Value"=w351:bool)  [unwired: 8 in, 2 out]
    n221 = call <vilib>:"WPI_DigitalInputGetValue.vi"("DigitalInputDevRef"=w353) -> ("Value"=w349:bool)  [unwired: 8 in, 2 out]
    n222 = call <vilib>:"WPI_DigitalInputGetValue.vi"("DigitalInputDevRef"=w359) -> ("Value"=w340:bool)  [unwired: 8 in, 2 out]
    n223 = call <vilib>:"WPI_DigitalInputGetValue.vi"("DigitalInputDevRef"=w358) -> ("Value"=w341:bool)  [unwired: 8 in, 2 out]
    n224 = call <vilib>:"WPI_DigitalInputGetValue.vi"("DigitalInputDevRef"=w360) -> ("Value"=w339:bool)  [unwired: 8 in, 2 out]
    n225 = call <vilib>:"WPI_DigitalInputGetValue.vi"("DigitalInputDevRef"=w361) -> ("Value"=w338:bool)  [unwired: 8 in, 2 out]
    n226 = Not(x=w339) -> (.not. x?=w345:bool)
    n227 = Not(x=w338) -> (.not. x?=w344:bool)
    n228 = Not(x=w341) -> (.not. x?=w347:bool)
    n229 = Not(x=w340) -> (.not. x?=w346:bool)
    n230 = Not(x=w343) -> (.not. x?=w342:bool)
    n231 = global write "Robot Global Data.vi" "fourbarBack"(w347) -> ()
    n232 = global write "Robot Global Data.vi" "lineLeftOn"(w351) -> ()
    n233 = global write "Robot Global Data.vi" "lineRightOn"(w349) -> ()
    n234 = global write "Robot Global Data.vi" "fourbarFwd"(w346) -> ()
    n235 = global write "Robot Global Data.vi" "dorsalDown"(w345) -> ()
    n236 = global write "Robot Global Data.vi" "lineCentOn"(w350) -> ()
    n237 = global write "Robot Global Data.vi" "cargo"(w342) -> ()
    n238 = global write "Robot Global Data.vi" "dorsalUp"(w344) -> ()
    n239 = Build Array(w344, w345, w346, w347, w351, w350, w349, w342) -> (w348:bool[])
    n240 = call-poly <vilib>:"NT Write Value.vi"("Boolean Array"=w348, "Name"="robotSensors") -> ()  [unwired: 9 in, 1 out]
    n241 = Wait (ms)(milliseconds to wait=u32 50) -> ()  [unwired: 1 out]
  }
  n242 = while {
    tunnel: w51 -> [w372]
    stop <- FALSE stop-if-true
    # "Shows you the integrated gyro outputs"
    # "Shows you the raw IMU outputs"
    # "Gyro Sensor"
    n243 = global read "Robot Global Data.vi" "Gyro Reset Deltas?"() -> (w370:bool)
    n244 = call "ADI_IMU_ADIS16470_Get Angles.vi"("ADI IMU DevRef"=w372) -> ("IMU Angles Out"=w368:T23)  [unwired: 7 in, 3 out]
    n245 = call "ADI_IMU_ADIS16470_Get Instant.vi"("ADI IMU DevRef"=w372) -> ("Sensor Ready Out"=w371:bool, "IMU Data"=w369:T24)  [unwired: 7 in, 2 out]
    n246 = case shown="True" w370 {
      tunnel: w372 -> [_ w376]
      frame False {
      }
      frame True {
        n247 = call "ADI_IMU_ADIS16470_Reset.vi"("ADI IMU DevRef"=w376) -> ()  [unwired: 9 in, 2 out]
        n248 = global write "Robot Global Data.vi" "Gyro Reset Deltas?"(FALSE) -> ()
      }
    }
    n249 = global write "Robot Global Data.vi" "IMU Angle Delta"(w368) -> ()
    n250 = global write "Robot Global Data.vi" "IMU Data"(w369) -> ()
    n251 = global write "Robot Global Data.vi" "Gyro Sensor Ready?"(w371) -> ()
    n252 = Unbundle(w368) -> ("X Angle"=w367:dbl, "Y Angle"=w366:dbl, "Z Angle"=w365:dbl)
    n253 = Build Array(w367, w366, w365) -> (w364:dbl[])
    n254 = call-poly <vilib>:"NT Write Value.vi"("Numeric Array"=w364, "Name"="gyroAngles") -> ()  [unwired: 9 in, 1 out]
    n255 = Wait (ms)(milliseconds to wait=u32 100) -> ()  [unwired: 1 out]
  }
